vi "Previous Step.vi"(8 "error in (no error)":errorcluster, 11 "ControlClassWizard in":refnum<class "QControl Creation Wizard.lvclass">) -> (0 "error out":errorcluster, 3 "ControlClassWizard out":refnum<class "QControl Creation Wizard.lvclass">)   [LabVIEW 2015, in "QControl Creation Wizard.lvclass"]
doc: "<b> </b> <b> </b>\n©2016 Q Software Innovations, LLC (QSI)\nwritten by Quentin Alldredge\nproduced in LabVIEW 2015\n\nsupport@qsoftwareinnovations.com\nwww.qsoftwareinnovations.com\n\nAll rights reserved.\n\nRedistribution and use in source and binary forms, with or without modification, are permitted provided that the following conditions are met:\n\n * Redistributions of source code must retain the above copyright notice, this list of conditions and the following disclaimer.\n * Redistributions in binary form must reproduce the above copyright notice, this list of conditions and the following disclaimer in the documentation and/or other materials provided with the distribution.\n * Neither the name of Q Software Innovations, LLC. nor the names of its contributors may be used to endorse or promote products derived from this software without specific prior written permission.\n\nTHIS SOFTWARE IS PROVIDED BY THE COPYRIGHT HOLDERS AND CONTRIBUTORS \"AS IS\" AND ANY EXPRESS OR IMPLIED WARRANTIES, INCLUDING, BUT NOT LIMITED TO, THE IMPLIED WARRANTIES OF MERCHANTABILITY AND FITNESS FOR A PARTICULAR PURPOSE ARE DISCLAIMED. IN NO EVENT SHALL THE COPYRIGHT OWNER OR CONTRIBUTORS BE LIABLE FOR ANY DIRECT, INDIRECT, INCIDENTAL, SPECIAL, EXEMPLARY, OR CONSEQUENTIAL DAMAGES (INCLUDING, BUT NOT LIMITED TO, PROCUREMENT OF SUBSTITUTE GOODS OR SERVICES; LOSS OF USE, DATA, OR PROFITS; OR BUSINESS INTERRUPTION) HOWEVER CAUSED AND ON ANY THEORY OF LIABILITY, WHETHER IN CONTRACT, STRICT LIABILITY, OR TORT (INCLUDING NEGLIGENCE OR OTHERWISE) ARISING IN ANY WAY OUT OF THE USE OF THIS SOFTWARE, EVEN IF ADVISED OF THE POSSIBILITY OF SUCH DAMAGE."
uses:
  QControl Creation Wizard.lvclass
  QControl Classes/Steps/Steps.lvclass
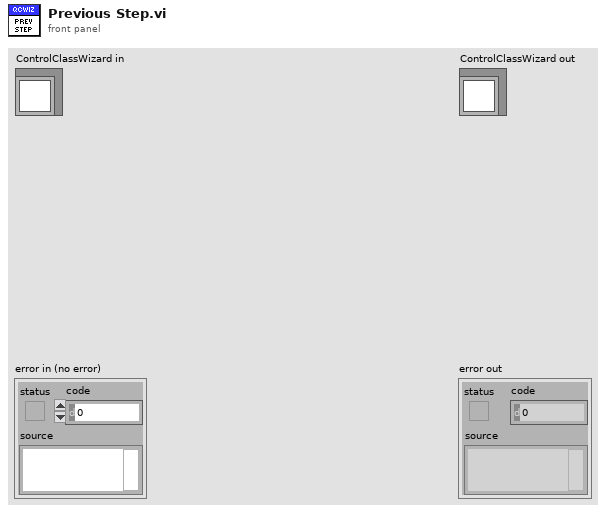
[diagram p1: front panel]
types:
  T1 = enum8{"Enabled", "Disabled", "Disabled and Grayed Out"}
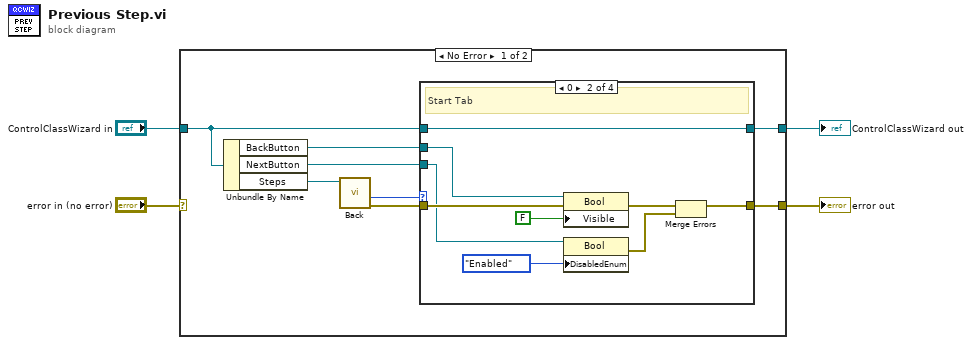
[diagram p0: block diagram]
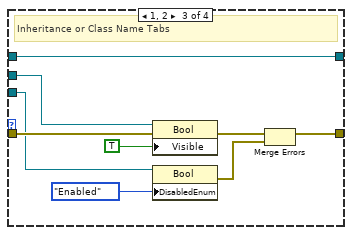
[diagram p3: hidden frame]
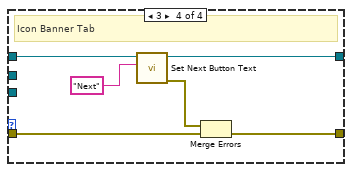
[diagram p4: hidden frame]
diagram:
  n1 = case shown="No Error" "error in (no error)" {
    selector: "error in (no error)" -> [_ w40]
    tunnel: [w7 w40] -> w3
    tunnel: [w5 w39] -> w1
    tunnel: "ControlClassWizard in" -> [w6 w39]
    frame No Error {
      n2 = Unbundle By Name(w6) -> ("BackButton"=w8:refnum<vi>, "NextButton"=w9:refnum<vi>, "Steps"=w12:refnum<class "Steps.lvclass">)
      n3 = call "Back.vi"("Steps in"=w12) -> ("error out"=w11:errorcluster, "Step Number"=w10:i32)  [unwired: 7 in, 2 out]
      n4 = case shown="0" w10 {
        tunnel: w11 -> [w14 w23 w32 w38]
        tunnel: [w14 w16 w25 w34] -> w7
        tunnel: w9 -> [_ w19 w28 _]
        tunnel: w8 -> [_ w21 w30 _]
        tunnel: w6 -> [w13 w17 w26 w36]
        tunnel: [w13 w17 w26 w35] -> w5
        frame Default {
        }
        frame 0 {
          # "Start Tab"
          n5 = property class="Bool"(reference=w21, error in=w23, "Visible"=FALSE ("Control:Visible")) -> (error out=w22:errorcluster)  [unwired: 1 out]
          n6 = property class="Bool"(reference=w19, "DisabledEnum"=T1."Enabled" ("Disabled")) -> (error out=w15:errorcluster)  [unwired: 1 in, 1 out]
          n7 = Merge Errors(w22, w15) -> (w16:errorcluster)
        }
        frame 1, 2 {
          # "Inheritance or Class Name Tabs"
          n8 = property class="Bool"(reference=w30, error in=w32, "Visible"=TRUE ("Control:Visible")) -> (error out=w31:errorcluster)  [unwired: 1 out]
          n9 = property class="Bool"(reference=w28, "DisabledEnum"=T1."Enabled" ("Disabled")) -> (error out=w24:errorcluster)  [unwired: 1 in, 1 out]
          n10 = Merge Errors(w31, w24) -> (w25:errorcluster)
        }
        frame 3 {
          # "Icon Banner Tab"
          n11 = call "Set Next Button Text.vi"("Text"="Next", "QControlWizard in"=w36) -> ("error out"=w33:errorcluster, "QControlWizard (dup)"=w35:refnum<class "QControl Creation Wizard.lvclass">)  [unwired: 8 in]
          n12 = Merge Errors(w33, w38) -> (w34:errorcluster)
        }
      }
    }
    frame Error {
    }
  }
  "error out" <- w3
  "ControlClassWizard out" <- w1
